vi "Init.vi"(8 "error in (no error)":errorcluster, 11 "Event_Syslog in":refnum<class "Event_Syslog.lvclass">) -> (0 "error out":errorcluster, 3 "Event_Syslog out":refnum<class "Event_Syslog.lvclass">)   [LabVIEW 2021, in "Event_Syslog.lvclass"]
uses:
  Event_Syslog.lvclass
  Event_Syslog.lvclass/Event_Syslog.ctl
  abs_EventLog/abs_EventLog.lvclass
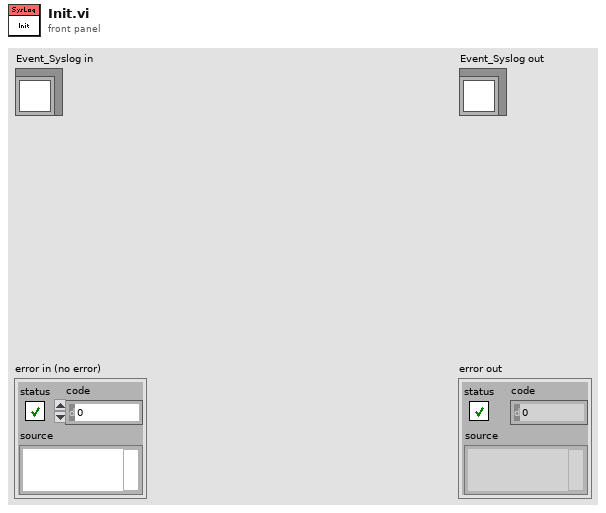
[diagram p1: front panel]
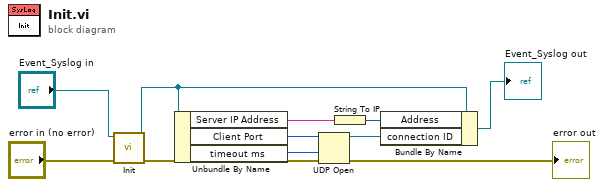
[diagram p0: block diagram]
diagram:
  n1 = call-parent "Init.vi"("error in (no error)"="error in (no error)", "abs_EventLog in"="Event_Syslog in") -> ("error out"=w9:errorcluster, "abs_EventLog out"=w4:refnum<class "Event_Syslog.lvclass">)  [unwired: 8 in]
  n2 = Unbundle By Name(w4) -> ("Server IP Address"=w3:string, "Client Port"=w2:u16, "timeout ms"=w1:i32)
  n3 = UDP Open(8:w9, 9:w1, 11:w2) -> (port=w5:refnum<k16>, 0:→"error out":errorcluster)  [unwired: 2 in, 1 out]
  n4 = String To IP(1:w3) -> (0:w6:u32)
  n5 = Bundle By Name(cluster=w4, "Address"=w6, "connection ID"=w5) -> (→"Event_Syslog out":refnum<class "Event_Syslog.lvclass">)
